vi "X_2500_X4.vi"(0 "x0":dbl format="%#_13g", 5 "x1":dbl format="%#_13g", 7 "x2":dbl format="%#_13g", 9 "x3":dbl format="%#_13g", 11 "x4":dbl format="%#_13g", 12 "e":dbl format="%#_13g", 13 "q0":dbl format="%#_13g", 14 "qzsum":dbl format="%#_13g") -> (8 "X4out":dbl)   [LabVIEW 2019]
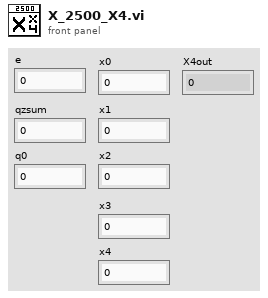
[diagram p1: front panel]
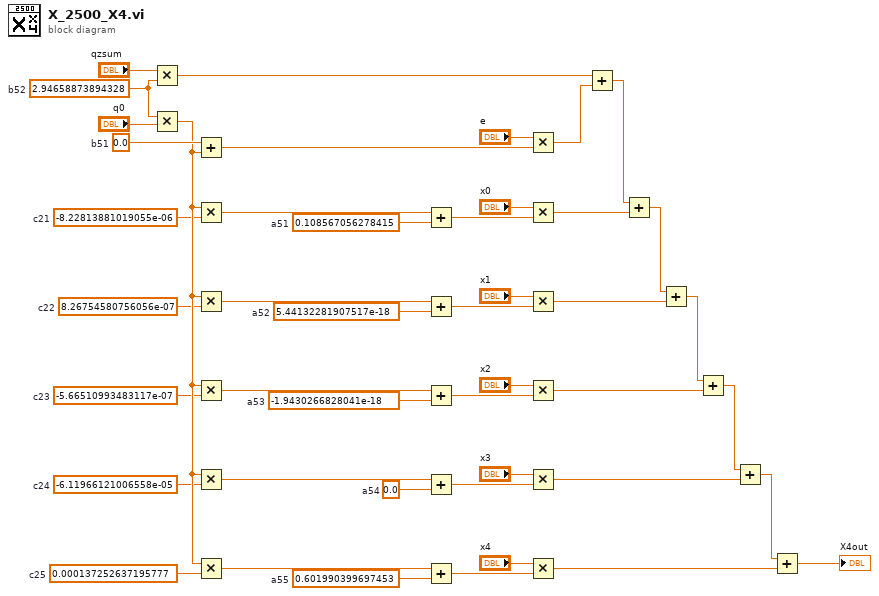
[diagram p0: block diagram]
diagram:
  w36 = 0.108567056278415  # a51
  w32 = -1.9430266828041e-18  # a53
  w28 = 0.601990399697453  # a55
  w30 = 0.0  # a54
  w34 = 5.44132281907517e-18  # a52
  w38 = -8.22813881019055e-06  # c21
  w40 = -5.66510993483117e-07  # c23
  w42 = 0.000137252637195777  # c25
  w41 = -6.11966121006558e-05  # c24
  w39 = 8.26754580756056e-07  # c22
  w7 = 2.94658873894328  # b52
  w44 = 0.0  # b51
  n1 = Multiply(x="qzsum", y=w7) -> (x*y=w4:dbl)
  n2 = Multiply(x=w7, y="q0") -> (x*y=w43:dbl)
  n3 = Add(x=w44, y=w43) -> (x+y=w2:dbl)
  n4 = Multiply(x=w43, y=w38) -> (x*y=w37:dbl)
  n5 = Multiply(x=w43, y=w39) -> (x*y=w35:dbl)
  n6 = Multiply(x=w43, y=w40) -> (x*y=w33:dbl)
  n7 = Multiply(x=w43, y=w41) -> (x*y=w31:dbl)
  n8 = Multiply(x=w43, y=w42) -> (x*y=w29:dbl)
  n9 = Add(x=w37, y=w36) -> (x+y=w24:dbl)
  n10 = Add(x=w35, y=w34) -> (x+y=w25:dbl)
  n11 = Add(x=w33, y=w32) -> (x+y=w26:dbl)
  n12 = Add(x=w31, y=w30) -> (x+y=w3:dbl)
  n13 = Add(x=w29, y=w28) -> (x+y=w27:dbl)
  n14 = Multiply(x="e", y=w2) -> (x*y=w5:dbl)
  n15 = Multiply(x="x0", y=w24) -> (x*y=w14:dbl)
  n16 = Multiply(x="x1", y=w25) -> (x*y=w13:dbl)
  n17 = Multiply(x="x2", y=w26) -> (x*y=w12:dbl)
  n18 = Multiply(x="x3", y=w3) -> (x*y=w11:dbl)
  n19 = Multiply(x="x4", y=w27) -> (x*y=w9:dbl)
  n20 = Add(x=w4, y=w5) -> (x+y=w16:dbl)
  n21 = Add(x=w16, y=w14) -> (x+y=w18:dbl)
  n22 = Add(x=w18, y=w13) -> (x+y=w15:dbl)
  n23 = Add(x=w15, y=w12) -> (x+y=w17:dbl)
  n24 = Add(x=w17, y=w11) -> (x+y=w10:dbl)
  n25 = Add(x=w10, y=w9) -> (x+y=→"X4out":dbl)
